vi "Master_DAQ_convertUnits.vi"(1 "Data Control In":T1={"cRIO Data"={"HallEffect Right (cm)"=0.0, "HallEffect Left (cm)"=0.0, "Optical Sensor 1 (V)"=0.0, "Optical Sensor 2 (V)"=0.0, "24V Voltage  (V)"=0.0, "24V Current (A)"=0.0, "Contactor H1 Continuity"=0.0, "Contactor L1 Continuity "=0.0, "Contactor H2 Continuity"=0.0, "Contactor L2 Continuity "=0.0, "Brake PT(psig)"=0.0, "Pump PT (psig)"=0.0, "24V Temp   (C)"=0.0, "Tank PT(psig) "=0.0, "ABS Pressure 1 (psig)"=0.0, "ABS Pressure 2 (psig) "=0.0, "Displacement (ft)"=0.0, "Velocity (ft/s)"=0.0, "Time (ms)"=0.0, "PV 1 Temp"=0.0, "PV2 Temp"=0.0}, "IMU Data"={"y acceleration (g)"=0.0, "Pressure (psia)"=0.0, "Temperature (F)"=0.0}, "BMS Data"={"Pack 1 Max Cell\n Voltage (V)"=0.0, "Pack 1 Max Cell\n ID "=0.0, "Pack 1 Min Cell \nVoltage (V)"=0.0, "Pack 1 Min Cell \nID "=0.0, "Pack 1 State of Charge  (%)"=0.0, "Pack 1 Average Voltage1 (V)"=0.0, "Pack 1Voltage Delta (V)"=0.0, "Pack 1 Current (A)"=0.0, "Pack 1 Voltage (V)"=0.0, "Pack 1 Max Resistance (Ohm)"=0.0, "Pack 1Min Resistance (Ohm)"=0.0, "Pack 1Average Resistance (Ohm)"=0.0, "Pack 1Delta Resistance (Ohm)"=0.0, "Pack 1 Highest Temperature(F)"=0.0, "BmsStatus1"={"isFault"=FALSE, "isolationMonitoring"=FALSE}, "Pack 2 Max Cell\n Voltage (V) "=0.0, "Pack 2 Max Cell\n ID  "=0.0, "Pack 2 Min Cell \nVoltage (V) "=0.0, "Pack 2 Min Cell \nID  "=0.0, "Pack 2 Average Voltage1 (V)"=0.0, "Pack 2 Voltage Delta (V) "=0.0, "Pack 2 Current (A)"=0.0, "Pack 2 Voltage (V) "=0.0, "Pack 2 State of Charge  (%) "=0.0, "Pack 2 Max Resistance (Ohm) "=0.0, "Pack 2 Min Resistance (Ohm)"=0.0, "Pack 2 Average Resistance (Ohm)"=0.0, "Pack 2 Delta Resistance (Ohm) "=0.0, "Pack 2 Highest Temperature(F) "=0.0, "BmsStatus 2"={"isFault"=FALSE, "isolationMonitoring"=FALSE}}, "Motor Data"={" Velocity (RPM)"=0.0, " MotorTemp(C)"=0.0, " ControlTemp(C)"=0.0, " DcLinkVolt(V)"=0.0, " ErrorCode"=0.0, "IsAlive"=FALSE, "motorStatus"={"isReady"=FALSE, "isOn"=FALSE, "isOperEn"=FALSE, "isFault"=FALSE, "isVoltEn"=FALSE, "targetReached"=FALSE, "isWarning"=FALSE}, "motorControllerState"=1}} {"Motor Data"."motorControllerState" items=["unknown"=1, "boot-up"=0, "stopped"=4, "operational"=5, "pre-operational"=127, "connection lost"=128]}) -> (0 "Data Out":T1={"cRIO Data"={"HallEffect Right (cm)"=0.0, "HallEffect Left (cm)"=0.0, "Optical Sensor 1 (V)"=0.0, "Optical Sensor 2 (V)"=0.0, "24V Voltage  (V)"=0.0, "24V Current (A)"=0.0, "Contactor H1 Continuity"=0.0, "Contactor L1 Continuity "=0.0, "Contactor H2 Continuity"=0.0, "Contactor L2 Continuity "=0.0, "Brake PT(psig)"=0.0, "Pump PT (psig)"=0.0, "24V Temp   (C)"=0.0, "Tank PT(psig) "=0.0, "ABS Pressure 1 (psig)"=0.0, "ABS Pressure 2 (psig) "=0.0, "Displacement (ft)"=0.0, "Velocity (ft/s)"=0.0, "Time (ms)"=0.0, "PV 1 Temp"=0.0, "PV2 Temp"=0.0}, "IMU Data"={"y acceleration (g)"=0.0, "Pressure (psia)"=0.0, "Temperature (F)"=0.0}, "BMS Data"={"Pack 1 Max Cell\n Voltage (V)"=0.0, "Pack 1 Max Cell\n ID "=0.0, "Pack 1 Min Cell \nVoltage (V)"=0.0, "Pack 1 Min Cell \nID "=0.0, "Pack 1 State of Charge  (%)"=0.0, "Pack 1 Average Voltage1 (V)"=0.0, "Pack 1Voltage Delta (V)"=0.0, "Pack 1 Current (A)"=0.0, "Pack 1 Voltage (V)"=0.0, "Pack 1 Max Resistance (Ohm)"=0.0, "Pack 1Min Resistance (Ohm)"=0.0, "Pack 1Average Resistance (Ohm)"=0.0, "Pack 1Delta Resistance (Ohm)"=0.0, "Pack 1 Highest Temperature(F)"=0.0, "BmsStatus1"={"isFault"=FALSE, "isolationMonitoring"=FALSE}, "Pack 2 Max Cell\n Voltage (V) "=0.0, "Pack 2 Max Cell\n ID  "=0.0, "Pack 2 Min Cell \nVoltage (V) "=0.0, "Pack 2 Min Cell \nID  "=0.0, "Pack 2 Average Voltage1 (V)"=0.0, "Pack 2 Voltage Delta (V) "=0.0, "Pack 2 Current (A)"=0.0, "Pack 2 Voltage (V) "=0.0, "Pack 2 State of Charge  (%) "=0.0, "Pack 2 Max Resistance (Ohm) "=0.0, "Pack 2 Min Resistance (Ohm)"=0.0, "Pack 2 Average Resistance (Ohm)"=0.0, "Pack 2 Delta Resistance (Ohm) "=0.0, "Pack 2 Highest Temperature(F) "=0.0, "BmsStatus 2"={"isFault"=FALSE, "isolationMonitoring"=FALSE}}, "Motor Data"={" Velocity (RPM)"=0.0, " MotorTemp(C)"=0.0, " ControlTemp(C)"=0.0, " DcLinkVolt(V)"=0.0, " ErrorCode"=0.0, "IsAlive"=FALSE, "motorStatus"={"isReady"=FALSE, "isOn"=FALSE, "isOperEn"=FALSE, "isFault"=FALSE, "isVoltEn"=FALSE, "targetReached"=FALSE, "isWarning"=FALSE}, "motorControllerState"=1}} {"Motor Data"."motorControllerState" items=["unknown"=1, "boot-up"=0, "stopped"=4, "operational"=5, "pre-operational"=127, "connection lost"=128]})   [LabVIEW 2018]
uses:
  Type_Def/Type_Def Master_DataControls.ctl
  Type_Def/TypeDef_cRIODatas.ctl
  Type_Def/Type_Def IMUDatas.ctl
  Type_Def/TypeDef_BMSDatas.ctl
  Type_Def/TypeDef_BMSStatuss.ctl
  Type_Def/TypeDef FixedMotorData.ctl
  Type_Def/TypeDef_MotorData.ctl
types:
  T1 = typedef "Type_Def Master_DataControls.ctl" = cluster{"cRIO Data":T2, "IMU Data":T3, "BMS Data":T4, "Motor Data":T6}
  T2 = typedef "TypeDef_cRIODatas.ctl" = cluster{"HallEffect Right (cm)":dbl, "HallEffect Left (cm)":dbl, "Optical Sensor 1 (V)":dbl, "Optical Sensor 2 (V)":dbl, "24V Voltage  (V)":dbl, "24V Current (A)":dbl, "Contactor H1 Continuity":dbl, "Contactor L1 Continuity ":dbl, "Contactor H2 Continuity":dbl, "Contactor L2 Continuity ":dbl, "Brake PT(psig)":dbl, "Pump PT (psig)":dbl, "24V Temp   (C)":dbl, "Tank PT(psig) ":dbl, "ABS Pressure 1 (psig)":dbl, "ABS Pressure 2 (psig) ":dbl, "Displacement (ft)":dbl, "Velocity (ft/s)":dbl, "Time (ms)":dbl, "PV 1 Temp":dbl, "PV2 Temp":dbl}
  T3 = typedef "Type_Def IMUDatas.ctl" = cluster{"y acceleration (g)":dbl, "Pressure (psia)":dbl, "Temperature (F)":dbl}
  T4 = typedef "TypeDef_BMSDatas.ctl" = cluster{"Pack 1 Max Cell\n Voltage (V)":dbl, "Pack 1 Max Cell\n ID ":dbl, "Pack 1 Min Cell \nVoltage (V)":dbl, "Pack 1 Min Cell \nID ":dbl, "Pack 1 State of Charge  (%)":dbl, "Pack 1 Average Voltage1 (V)":dbl, "Pack 1Voltage Delta (V)":dbl, "Pack 1 Current (A)":dbl, "Pack 1 Voltage (V)":dbl, "Pack 1 Max Resistance (Ohm)":dbl, "Pack 1Min Resistance (Ohm)":dbl, "Pack 1Average Resistance (Ohm)":dbl, "Pack 1Delta Resistance (Ohm)":dbl, "Pack 1 Highest Temperature(F)":dbl, "BmsStatus1":T5, "Pack 2 Max Cell\n Voltage (V) ":dbl, "Pack 2 Max Cell\n ID  ":dbl, "Pack 2 Min Cell \nVoltage (V) ":dbl, "Pack 2 Min Cell \nID  ":dbl, "Pack 2 Average Voltage1 (V)":dbl, "Pack 2 Voltage Delta (V) ":dbl, "Pack 2 Current (A)":dbl, "Pack 2 Voltage (V) ":dbl, "Pack 2 State of Charge  (%) ":dbl, "Pack 2 Max Resistance (Ohm) ":dbl, "Pack 2 Min Resistance (Ohm)":dbl, "Pack 2 Average Resistance (Ohm)":dbl, "Pack 2 Delta Resistance (Ohm) ":dbl, "Pack 2 Highest Temperature(F) ":dbl, "BmsStatus 2":T5}
  T5 = typedef "TypeDef_BMSStatuss.ctl" = cluster{"isFault":bool, "isolationMonitoring":bool}
  T6 = typedef "TypeDef FixedMotorData.ctl" = cluster{" Velocity (RPM)":dbl, " MotorTemp(C)":dbl, " ControlTemp(C)":dbl, " DcLinkVolt(V)":dbl, " ErrorCode":dbl, "IsAlive":bool, "motorStatus":cluster{"isReady":bool, "isOn":bool, "isOperEn":bool, "isFault":bool, "isVoltEn":bool, "targetReached":bool, "isWarning":bool}, "motorControllerState":u16}
  T7 = typedef "TypeDef_MotorData.ctl" = cluster{" Velocity (RPM)":i32, " MotorTemp(C)":u8, " ControlTemp(C)":u8, " DcLinkVolt(V)":dbl, " ErrorCode":dbl, "IsAlive":bool, "motorStatus":cluster{"isReady":bool, "isOn":bool, "isOperEn":bool, "isFault":bool, "isVoltEn":bool, "targetReached":bool, "isWarning":bool}, "motorControllerState":u16}
  T8 = cluster{"isReady":bool, "isOn":bool, "isOperEn":bool, "isFault":bool, "isVoltEn":bool, "targetReached":bool, "isWarning":bool}
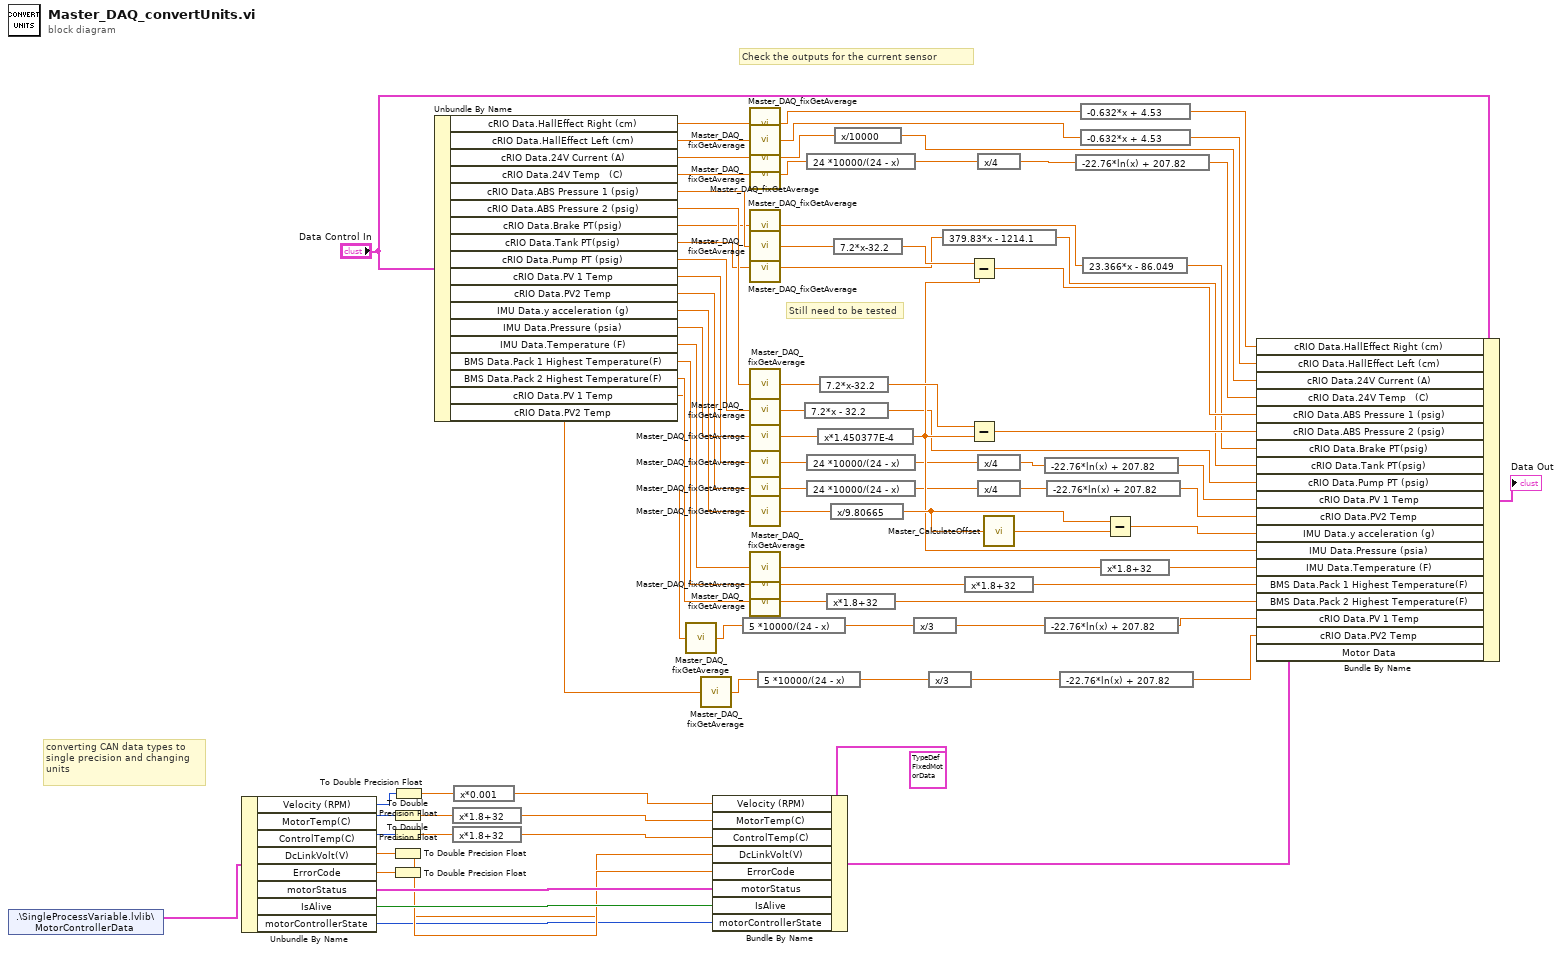
[diagram p0: block diagram]
diagram:
  # "Check the outputs for the current sensor"
  # "Still need to be tested"
  # "converting CAN data types to\nsingle precision and changing\nunits"
  n1 = shared-variable ".\\SingleProcessVariable.lvlib\\MotorControllerData"() -> (w71:T7)  [unwired: 1 in, 1 out]
  n2 = Unbundle By Name(w71) -> ("Velocity (RPM)"=w89:i32, "MotorTemp(C)"=w87:u8, "ControlTemp(C)"=w86:u8, "DcLinkVolt(V)"=w85:dbl, "ErrorCode"=w84:dbl, "motorStatus"=w82:T8, "IsAlive"=w83:bool, "motorControllerState"=w72:u16)
  n3 = To Double Precision Float(number=w87) -> (double precision float=w75:dbl)
  n4 = To Double Precision Float(number=w86) -> (double precision float=w79:dbl)
  n5 = To Double Precision Float(number=w85) -> (double precision float=w77:dbl)
  n6 = To Double Precision Float(number=w84) -> (double precision float=w78:dbl)
  n7 = To Double Precision Float(number=w89) -> (double precision float=w81:dbl)
  n8 = Unbundle By Name("Data Control In") -> ("cRIO Data.HallEffect Right (cm)"=w64:dbl, "cRIO Data.HallEffect Left (cm)"=w63:dbl, "cRIO Data.24V Current (A)"=w62:dbl, "cRIO Data.24V Temp   (C)"=w61:dbl, "cRIO Data.ABS Pressure 1 (psig)"=w60:dbl, "cRIO Data.ABS Pressure 2 (psig)"=w59:dbl, "cRIO Data.Brake PT(psig)"=w58:dbl, "cRIO Data.Tank PT(psig)"=w57:dbl, "cRIO Data.Pump PT (psig)"=w56:dbl, "cRIO Data.PV 1 Temp"=w20:dbl, "cRIO Data.PV2 Temp"=w19:dbl, "IMU Data.y acceleration (g)"=w55:dbl, "IMU Data.Pressure (psia)"=w54:dbl, "IMU Data.Temperature (F)"=w53:dbl, "BMS Data.Pack 1 Highest Temperature(F)"=w52:dbl, "BMS Data.Pack 2 Highest Temperature(F)"=w51:dbl, "cRIO Data.PV 1 Temp"=w10:dbl, "cRIO Data.PV2 Temp"=w1:dbl)
  n9 = expression code="x*1.8+32"(w75) -> (w74:dbl)
  n10 = expression code="x*1.8+32"(w79) -> (w76:dbl)
  n11 = expression code="x*0.001"(w81) -> (w80:dbl)
  n12 = call "Master_DAQ_fixGetAverage.vi"("new value"=w10) -> ("mean"=w9:dbl)
  n13 = call "Master_DAQ_fixGetAverage.vi"("new value"=w1) -> ("mean"=w2:dbl)
  n14 = Bundle By Name(cluster=T6 {" Velocity (RPM)"=0.0, " MotorTemp(C)"=0.0, " ControlTemp(C)"=0.0, " DcLinkVolt(V)"=0.0, " ErrorCode"=0.0, "IsAlive"=FALSE, "motorStatus"={"isReady"=FALSE, "isOn"=FALSE, "isOperEn"=FALSE, "isFault"=FALSE, "isVoltEn"=FALSE, "targetReached"=FALSE, "isWarning"=FALSE}, "motorControllerState"=1} ("motorData"), "Velocity (RPM)"=w80, "MotorTemp(C)"=w74, "ControlTemp(C)"=w76, "DcLinkVolt(V)"=w77, "ErrorCode"=w78, "motorStatus"=w82, "IsAlive"=w83, "motorControllerState"=w72) -> (w73:T6)
  n15 = expression code="5 *10000/(24 - x)"(w9) -> (w8:dbl)
  n16 = call "Master_DAQ_fixGetAverage.vi"("new value"=w64) -> ("mean"=w50:dbl)
  n17 = call "Master_DAQ_fixGetAverage.vi"("new value"=w63) -> ("mean"=w49:dbl)
  n18 = call "Master_DAQ_fixGetAverage.vi"("new value"=w62) -> ("mean"=w42:dbl)
  n19 = call "Master_DAQ_fixGetAverage.vi"("new value"=w61) -> ("mean"=w41:dbl)
  n20 = call "Master_DAQ_fixGetAverage.vi"("new value"=w58) -> ("mean"=w39:dbl)
  n21 = call "Master_DAQ_fixGetAverage.vi"("new value"=w60) -> ("mean"=w40:dbl)
  n22 = call "Master_DAQ_fixGetAverage.vi"("new value"=w57) -> ("mean"=w38:dbl)
  n23 = call "Master_DAQ_fixGetAverage.vi"("new value"=w59) -> ("mean"=w48:dbl)
  n24 = call "Master_DAQ_fixGetAverage.vi"("new value"=w56) -> ("mean"=w37:dbl)
  n25 = call "Master_DAQ_fixGetAverage.vi"("new value"=w54) -> ("mean"=w44:dbl)
  n26 = call "Master_DAQ_fixGetAverage.vi"("new value"=w20) -> ("mean"=w14:dbl)
  n27 = call "Master_DAQ_fixGetAverage.vi"("new value"=w19) -> ("mean"=w13:dbl)
  n28 = call "Master_DAQ_fixGetAverage.vi"("new value"=w55) -> ("mean"=w43:dbl)
  n29 = call "Master_DAQ_fixGetAverage.vi"("new value"=w53) -> ("mean"=w45:dbl)
  n30 = call "Master_DAQ_fixGetAverage.vi"("new value"=w52) -> ("mean"=w46:dbl)
  n31 = call "Master_DAQ_fixGetAverage.vi"("new value"=w51) -> ("mean"=w47:dbl)
  n32 = expression code="5 *10000/(24 - x)"(w2) -> (w3:dbl)
  n33 = expression code="7.2*x - 32.2"(w37) -> (w24:dbl)
  n34 = expression code="24 *10000/(24 - x)"(w41) -> (w23:dbl)
  n35 = expression code="24 *10000/(24 - x)"(w14) -> (w17:dbl)
  n36 = expression code="24 *10000/(24 - x)"(w13) -> (w16:dbl)
  n37 = expression code="x*1.450377E-4"(w44) -> (w28:dbl)
  n38 = expression code="7.2*x-32.2"(w48) -> (w68:dbl)
  n39 = expression code="x*1.8+32"(w47) -> (w25:dbl)
  n40 = expression code="x/9.80665"(w43) -> (w65:dbl)
  n41 = expression code="7.2*x-32.2"(w40) -> (w67:dbl)
  n42 = expression code="x/10000"(w42) -> (w34:dbl)
  n43 = expression code="x/3"(w8) -> (w7:dbl)
  n44 = expression code="x/3"(w3) -> (w4:dbl)
  n45 = expression code="379.83*x - 1214.1"(w38) -> (w30:dbl)
  n46 = expression code="x*1.8+32"(w46) -> (w26:dbl)
  n47 = Subtract(x=w67, y=w28) -> (x-y=w33:dbl)
  n48 = Subtract(x=w68, y=w28) -> (x-y=w32:dbl)
  n49 = expression code="x/4"(w23) -> (w21:dbl)
  n50 = expression code="x/4"(w17) -> (w18:dbl)
  n51 = expression code="x/4"(w16) -> (w15:dbl)
  n52 = call "Master_CalculateOffset.vi"("Acceleration"=w65) -> ("Offset"=w66:dbl)
  n53 = expression code="-22.76*ln(x) + 207.82"(w18) -> (w12:dbl)
  n54 = expression code="-22.76*ln(x) + 207.82"(w7) -> (w6:dbl)
  n55 = expression code="-22.76*ln(x) + 207.82"(w15) -> (w11:dbl)
  n56 = expression code="-22.76*ln(x) + 207.82"(w4) -> (w5:dbl)
  n57 = expression code="-22.76*ln(x) + 207.82"(w21) -> (w22:dbl)
  n58 = expression code="-0.632*x + 4.53"(w50) -> (w36:dbl)
  n59 = expression code="-0.632*x + 4.53"(w49) -> (w35:dbl)
  n60 = expression code="23.366*x - 86.049"(w39) -> (w31:dbl)
  n61 = expression code="x*1.8+32"(w45) -> (w27:dbl)
  n62 = Subtract(x=w65, y=w66) -> (x-y=w29:dbl)
  n63 = Bundle By Name(cluster="Data Control In", "cRIO Data.HallEffect Right (cm)"=w36, "cRIO Data.HallEffect Left (cm)"=w35, "cRIO Data.24V Current (A)"=w34, "cRIO Data.24V Temp   (C)"=w22, "cRIO Data.ABS Pressure 1 (psig)"=w33, "cRIO Data.ABS Pressure 2 (psig)"=w32, "cRIO Data.Brake PT(psig)"=w31, "cRIO Data.Tank PT(psig)"=w30, "cRIO Data.Pump PT (psig)"=w24, "cRIO Data.PV 1 Temp"=w12, "cRIO Data.PV2 Temp"=w11, "IMU Data.y acceleration (g)"=w29, "IMU Data.Pressure (psia)"=w28, "IMU Data.Temperature (F)"=w27, "BMS Data.Pack 1 Highest Temperature(F)"=w26, "BMS Data.Pack 2 Highest Temperature(F)"=w25, "cRIO Data.PV 1 Temp"=w6, "cRIO Data.PV2 Temp"=w5, "Motor Data"=w73) -> (→"Data Out":T1)
